vi "MDAQ_CollectSurfaceSpectrum.vi"(9 "Cluster IN":T1 {"CV"."Temperature Array" scale=0.0..100.0}, 10 "Status Cluster In":T3 {"GATESTOP" format="%04x"; "GATESTRT" format="%04x"; "AMPLITUDE" format="%04x"; "M_CYCLES" format="%04x"; "N_CYCLES" format="%04x"; "STEP" format="%04x"; "BASE" format="%04x"; "CHAN" format="%04x"}, 11 "CurrectSpectrum":u32[](array[numeric])) -> (1 "Cluster Out":T1 {"CV"."Temperature Array" scale=0.0..100.0}, 2 "Status Cluster Out":T3 {"GATESTOP" format="%04x"; "GATESTRT" format="%04x"; "AMPLITUDE" format="%04x"; "M_CYCLES" format="%04x"; "N_CYCLES" format="%04x"; "STEP" format="%04x"; "BASE" format="%04x"; "CHAN" format="%04x"})   [LabVIEW 2021]
uses:
  Status_Cluster.ctl
  GUI_Def.ctl
  Mode_Enum.ctl
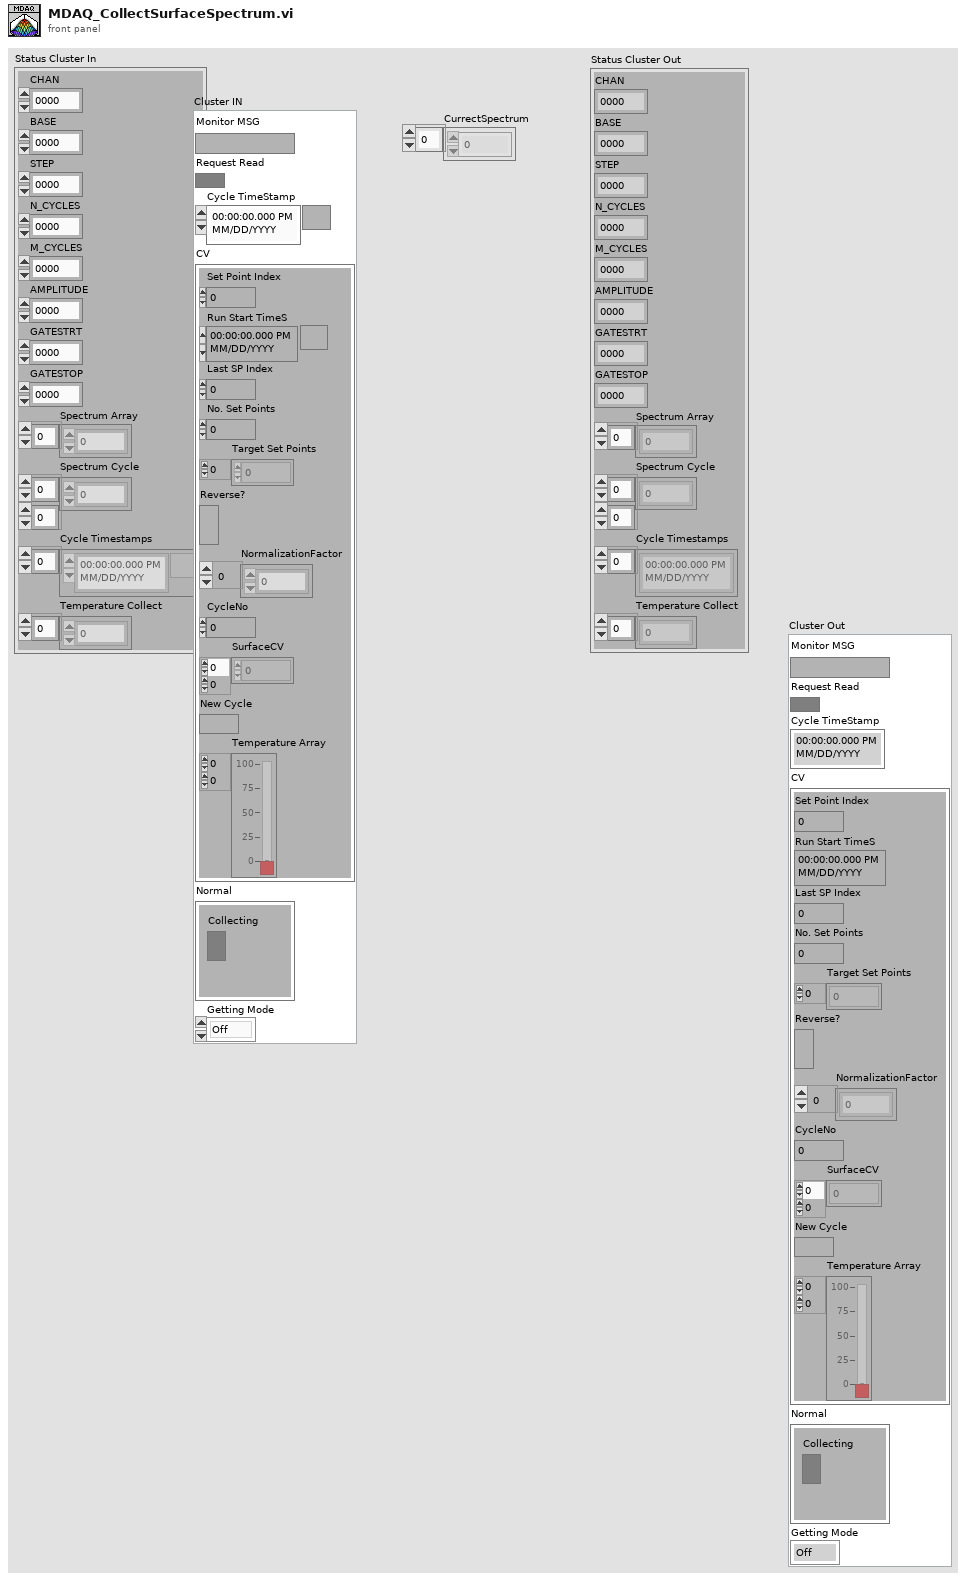
[diagram p1: front panel]
types:
  T1 = typedef "GUI_Def.ctl" = cluster{"Monitor MSG":string, "Request Read":bool, "Cycle TimeStamp":timestamp, "CV":cluster{"Set Point Index":u32, "Run Start TimeS":timestamp, "Last SP Index":u32, "No. Set Points":u32, "Target Set Points":i32[], "Reverse?":bool, "NormalizationFactor":i32[], "CycleNo":i32, "SurfaceCV":dbl[][], "New Cycle":bool, "Temperature Array":dbl[][]}, "Normal":cluster{"Collecting":bool}, "Getting Mode":T2}
  T2 = typedef "Mode_Enum.ctl" = enum16{"Off", "Normal", "CV+Temp", "CV"}
  T3 = typedef "Status_Cluster.ctl" = cluster{"CHAN":u32, "BASE":u32, "STEP":u32, "N_CYCLES":u32, "M_CYCLES":u32, "AMPLITUDE":u32, "GATESTRT":u32, "GATESTOP":u32, "Spectrum Array":u32[], "Spectrum Cycle":u32[][], "Cycle Timestamps":timestamp[], "Temperature Collect":dbl[]}
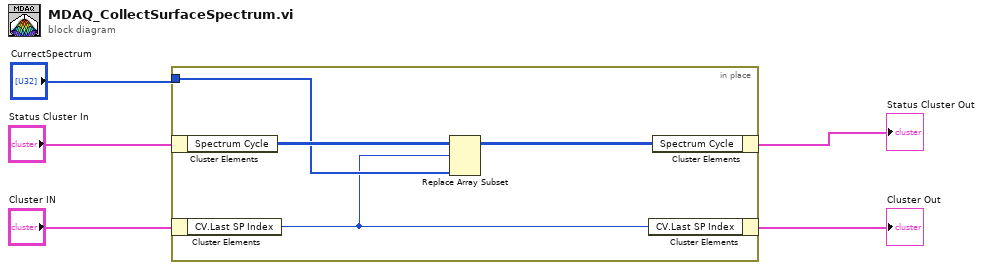
[diagram p0: block diagram]
diagram:
  n1 = in-place {
    in-place-border: "CurrectSpectrum" -> [w8]
    n2 = in-place-cluster #1("Status Cluster In") -> ("Spectrum Cycle"=w9:u32[][])
    n3 = in-place-cluster #2("Cluster IN") -> ("CV.Last SP Index"=w6:u32)
    n4 = Replace Array Subset(array=w9, new element=w8, index (row)=w6) -> (w7:u32[][])  [unwired: 1 in]
    n5 = in-place-cluster #2("CV.Last SP Index"=w6) -> (→"Cluster Out":T1)
    n6 = in-place-cluster #1("Spectrum Cycle"=w7) -> (→"Status Cluster Out":T3)
  }
